vi "clusterarrayformula.vi"() -> ()   [LabVIEW 2022 SP3]
panel:
  out "Final Array":dbl[](array[numeric])
  in  "stop":bool
  out "5th element":dbl
  out "New Array":dbl[](array[numeric])
  in  "Original Array":dbl[](array[numeric])
  in  "Cluster":cluster{"x":dbl, "index":dbl, "y":dbl}
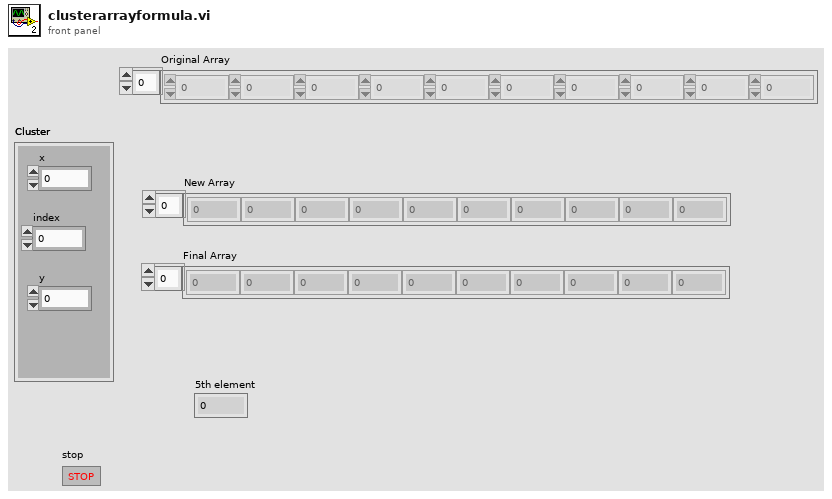
[diagram p1: front panel]
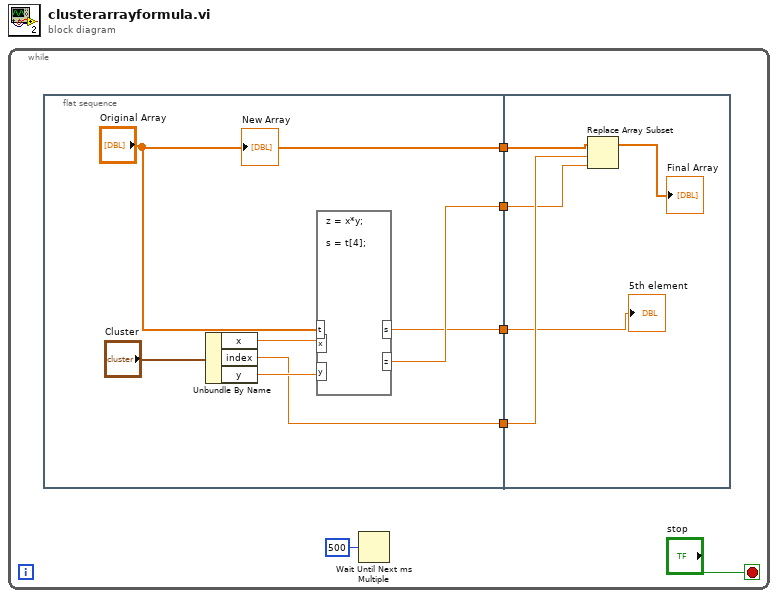
[diagram p0: block diagram]
diagram:
  n1 = while {
    stop <- "stop" stop-if-true
    n2 = flat-sequence {
      tunnel: ["Original Array"] -> w6
      tunnel: [w10] -> w5
      tunnel: [w9] -> w4
      tunnel: [w7] -> w3
      tunnel: w6 -> [w16]
      tunnel: w5 -> [w17]
      tunnel: w4 -> [w18]
      tunnel: w3 -> [w15]
      frame #0 {
        n3 = Unbundle By Name("Cluster") -> ("x"=w12:dbl, "index"=w9:dbl, "y"=w11:dbl)
        n4 = formula code="z = x*y;\n\ns = t[4];"("x"=w12, "y"=w11, "t"="Original Array") -> ("z"=w10:dbl, "s"=w7:dbl)
        "New Array" <- "Original Array"
      }
      frame #1 {
        n5 = Replace Array Subset "Replace Array Subset"(array=w16, new element=w17, index=w18) -> (→"Final Array":dbl[])
        "5th element" <- w15
      }
    }
    n6 = Wait Until Next ms Multiple(millisecond multiple=u32 500) -> ()  [unwired: 1 out]
  }
